vi "CRYWaveform Autosave.vi"(9 "File path":path, 11 "Flatten Wave":string[](array[string])) -> ()   [LabVIEW 2013]
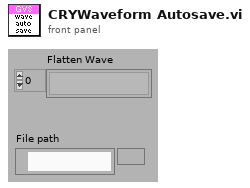
[diagram p1: front panel]
types:
  T1 = typedef "CRYWaveform Cluster.ctl" = cluster{"Waveform":cluster{"X0":dbl, "dX":dbl, "Y":sgl[]}, "X data":u16, "Y data":u16, "Y axis":u16, "X unit":string, "Y unit":string, "Y dB ref":dbl, "display Y":bool, "display X":bool, "Overload?":bool, "Test Info":string, "Step No.":i32, "Name":string, "protected":bool, "Sqc history":string[], "Signal Channel ID":i32, "Plot Settings":cluster{"Color":u32, "Interpolation":u8, "Point Style":u8, "Line Style":u8, "Point Color":u32, "Line Width":u8, "Bar Plot Style":u8, "Fill To":i16}, "AutoProtect":bool}
  T2 = enum16{"OK", "Yes", "YesNo", "YesNoCancel", "ReplaceAppend"}
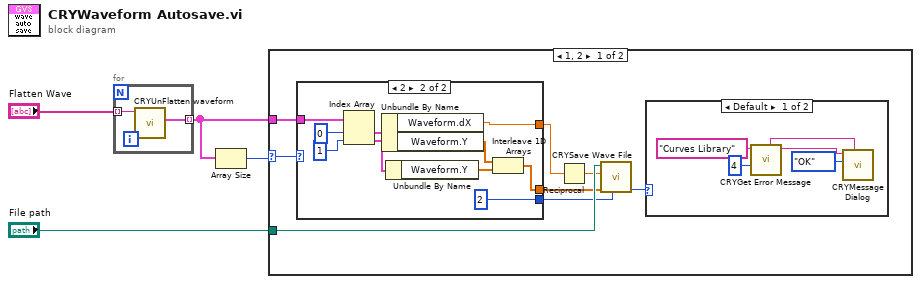
[diagram p0: block diagram]
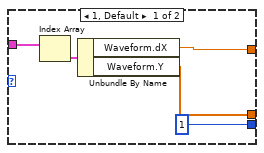
[diagram p3: hidden frame]
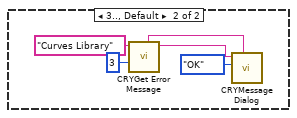
[diagram p4: hidden frame]
diagram:
  n1 = for {
    tunnel: "Flatten Wave" -> [w6] mode=indexing
    tunnel: [w5] -> w1 mode=indexing
    n2 = call "CRYUnFlatten waveform.vi"("Unflatten Waveform"=w6) -> ("Waveform Cluster"=w5:T1)  [unwired: 8 in, 2 out]
  }
  n3 = Array Size(array=w1) -> (size(s)=w3:i32)
  n4 = case shown="1, 2" w3 {
    selector: w3 -> [w10 _]
    tunnel: w1 -> [w11 _]
    tunnel: "File path" -> [w13 _]
    frame 1, 2 {
      n5 = case shown="2" w10 {
        tunnel: [w23 w33] -> w14
        tunnel: w11 -> [w22 w32]
        tunnel: [w21 w29] -> w9
        tunnel: [u32 1 ("Channel") u32 2 ("Channel")] -> w7
        frame 1, Default {
          n6 = Index Array(array=w22) -> (element=w24:T1)  [unwired: 1 in]
          n7 = Unbundle By Name(w24) -> ("Waveform.dX"=w23:dbl, "Waveform.Y"=w21:sgl[])
        }
        frame 2 {
          n8 = Index Array(array=w32, index #1=0 ("index"), index #2=1 ("index")) -> (element #1=w34:T1, element #2=w27:T1)
          n9 = Unbundle By Name(w34) -> ("Waveform.dX"=w33:dbl, "Waveform.Y"=w31:sgl[])
          n10 = Unbundle By Name(w27) -> ("Waveform.Y"=w30:sgl[])
          n11 = Interleave 1D Arrays(w31, w30) -> (w29:sgl[])
        }
      }
      n12 = Reciprocal(x=w14) -> (1/x=w12:dbl)
      n13 = call "CRYSave Wave File.vi"("Channel"=w7, "Wave Data In"=w9, "Sampling Freq"=w12, "Wave File Path In"=w13) -> ("Error Out(0-OK)"=w8:u32)  [unwired: 7 in]
      n14 = case shown="Default" w8 {
        frame Default {
          n15 = call "CRYGet Error Message.vi"("Error No"=4, "Kind"="Curves Library") -> ("Message"=w16:string, "Window Title"=w15:string)  [unwired: 4 in, 4 out]
          n16 = call "CRYMessage Dialog.vi"("Window Title"=w15, "YesNoCancel"=T2."OK", "Message Content"=w16) -> ()  [unwired: 7 in, 2 out]
        }
        frame 0 {
        }
      }
    }
    frame 3.., Default {
      n17 = call "CRYGet Error Message.vi"("Error No"=3, "Kind"="Curves Library") -> ("Message"=w35:string, "Window Title"=w36:string)  [unwired: 4 in, 4 out]
      n18 = call "CRYMessage Dialog.vi"("Window Title"=w36, "YesNoCancel"=T2."OK", "Message Content"=w35) -> ()  [unwired: 7 in, 2 out]
    }
  }
